vi "read.vi"(8 "error in (no error)":errorcluster, 11 "Device in":T1) -> (0 "error out":errorcluster, 2 "data":string, 3 "Device out":T1)   [LabVIEW 2016]
uses:
  device.ctl
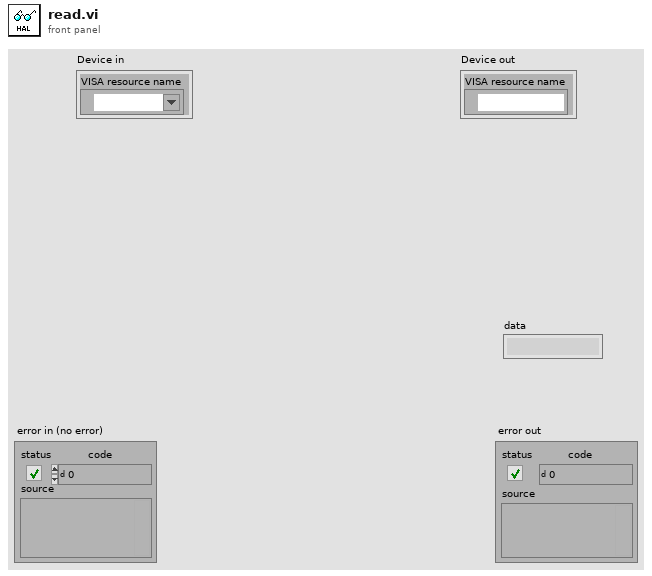
[diagram p1: front panel]
types:
  T1 = typedef "device.ctl" = cluster{"VISA resource name":refnum<visa-resource-name>}
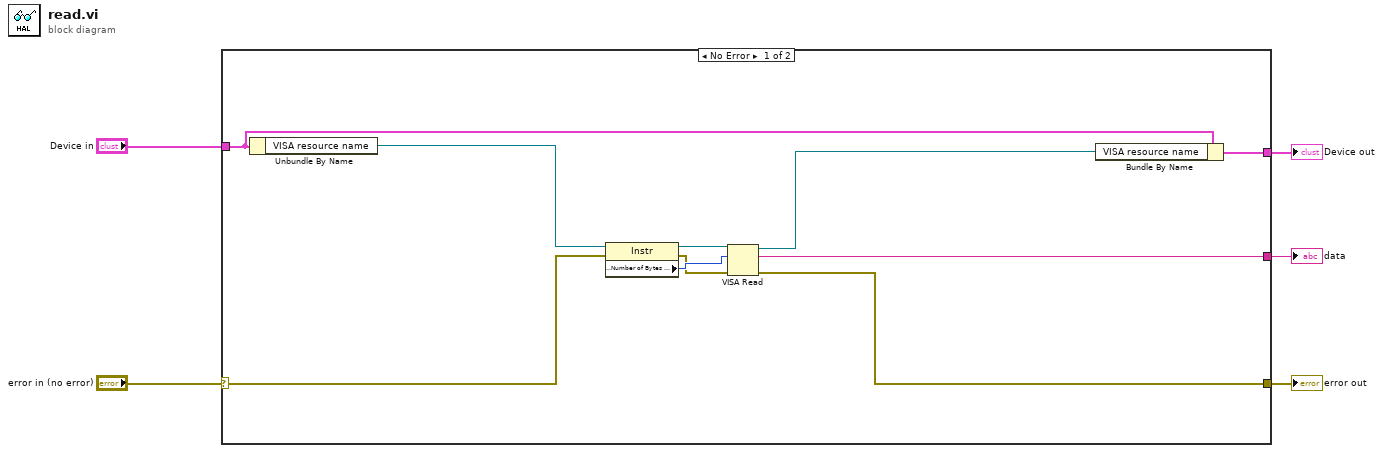
[diagram p0: block diagram]
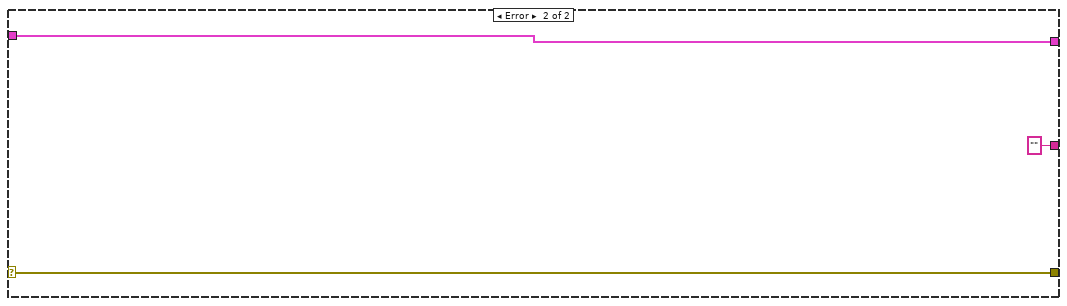
[diagram p2: hidden frame]
diagram:
  n1 = case shown="No Error" "error in (no error)" {
    selector: "error in (no error)" -> [w15 w17]
    tunnel: [w7 w18] -> w4
    tunnel: "Device in" -> [w8 w18]
    tunnel: [w14 w17] -> w2
    tunnel: [w12 "" ("read buffer")] -> w1
    frame No Error {
      n2 = Unbundle By Name(w8) -> ("VISA resource name"=w6:refnum<visa-resource-name>)
      n3 = property class="Instr"(reference=w6, error in=w15) -> (reference out=w9:refnum<visa-resource-name>, error out=w10:errorcluster, "Serial Settings:Number of Bytes at Serial Port"=w11:u32)
      n4 = VISA Read(VISA resource name=w9, byte count=w11, error in (no error)=w10) -> (VISA resource name out=w13:refnum<visa-resource-name>, read buffer=w12:string, error out=w14:errorcluster)  [unwired: 1 out]
      n5 = Bundle By Name(cluster=w8, "VISA resource name"=w13) -> (w7:T1)
    }
    frame Error {
    }
  }
  "error out" <- w2
  "Device out" <- w4
  "data" <- w1
